vi "TcpIP_Server.vi"() -> ()   [LabVIEW 2011]
uses:
  <vilib>/Utility/file.llb/Write To Spreadsheet File (string).vi
panel:
  out "数据输出 2":string
  in  "停止 2":bool
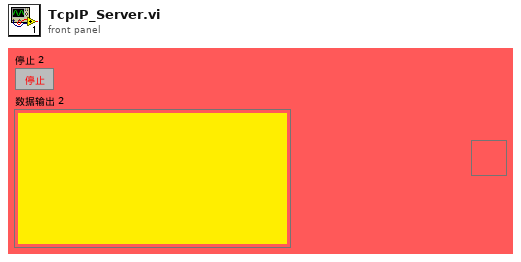
[diagram p1: front panel]
types:
  T1 = enum16{"Standard", "Buffered", "CRLF", "Immediate"}
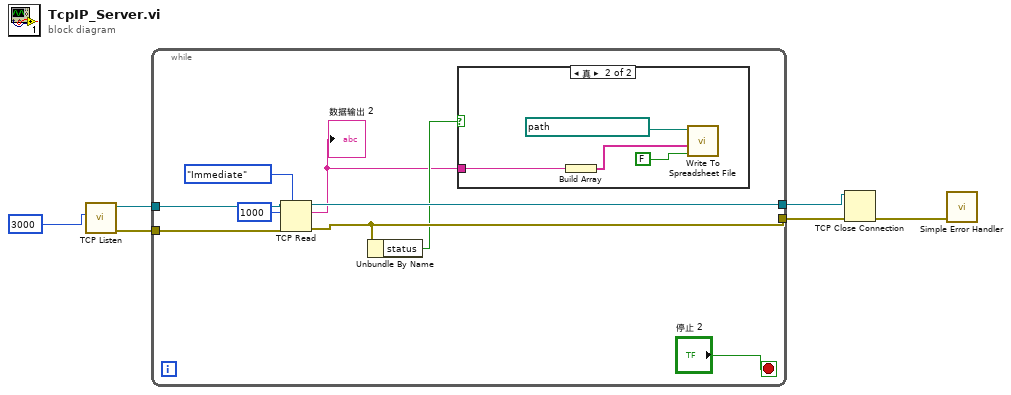
[diagram p0: block diagram]
diagram:
  n1 = call <vilib>:"TCP Listen.vi"("port"=3000 ("timeout ms (wait forever: -1)")) -> ("error out"=w4:errorcluster, "connection ID"=w3:refnum<k5>)  [unwired: 6 in, 3 out]
  n2 = while {
    tunnel: [w9] -> w5
    tunnel: w4 -> [w14]
    tunnel: w3 -> [w13]
    tunnel: [w10] -> w2
    stop <- "停止 2" stop-if-true
    n3 = TCP Read(connection ID=w13, bytes to read=1000 ("读取的字节"), error in (no error)=w14, 7:T1."Immediate" ("模式（标准）")) -> (connection ID out=w10:refnum<k5>, data out=w7:string, error out=w9:errorcluster)  [unwired: 1 in]
    "数据输出 2" <- w7
    n4 = Unbundle By Name(w9) -> ("status"=w8:bool)
    n5 = case shown="真" w8 {
      tunnel: w7 -> [_ w19]
      frame False {
      }
      frame True {
        n6 = Build Array(w19) -> (w17:string[])
        n7 = call-poly <vilib>:"Write To Spreadsheet File.vi"("append to file? (new file:F)"=FALSE, "1D data"=w17, "file path (dialog if empty)"=path "D:/Users/Administrator/Desktop/新文字文件.txt") -> ()  [unwired: 5 in, 1 out]
      }
    }
  }
  n8 = TCP Close Connection(connection ID=w2, error in (no error)=w5) -> (error out=w6:errorcluster)  [unwired: 1 in, 1 out]
  n9 = call <vilib>:"Simple Error Handler.vi"("error in (no error)"=w6) -> ()  [unwired: 4 in, 5 out]
